vi "Field to Voltage 1D.vi"(11 "Magnetic field [µT]":dbl) -> ()   [LabVIEW 2018]
panel:
  out "Voltage X":string
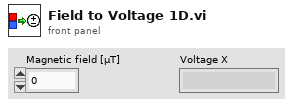
[diagram p1: front panel]
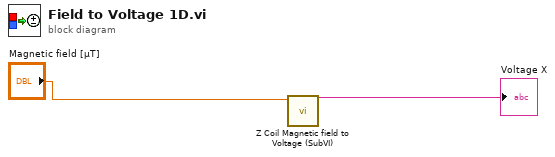
[diagram p0: block diagram]
diagram:
  n1 = call "Z Coil Magnetic field to Voltage (SubVI).vi"("Magnetic field [µT]"="Magnetic field [µT]") -> ("Voltage X"=→"Voltage X":string)  [unwired: 10 in]
